vi "Temperature load wafer counts.vi"() -> ()   [LabVIEW 2015, in "VIPM2.lvlib"]
uses:
  VIPM2.lvlib
panel:
  out "Wafer counts":sgl[](array[numeric]) format="%.1f"
  out "ChipIDs":u16[](array[numeric]) format="%04x"
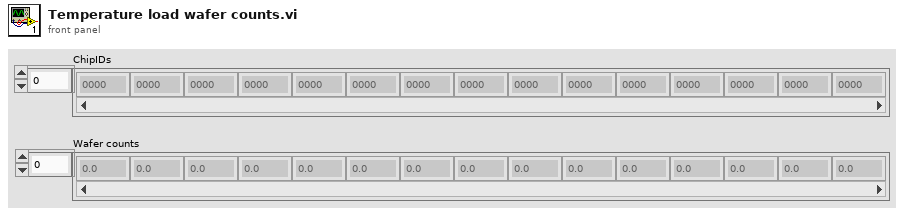
[diagram p1: front panel]
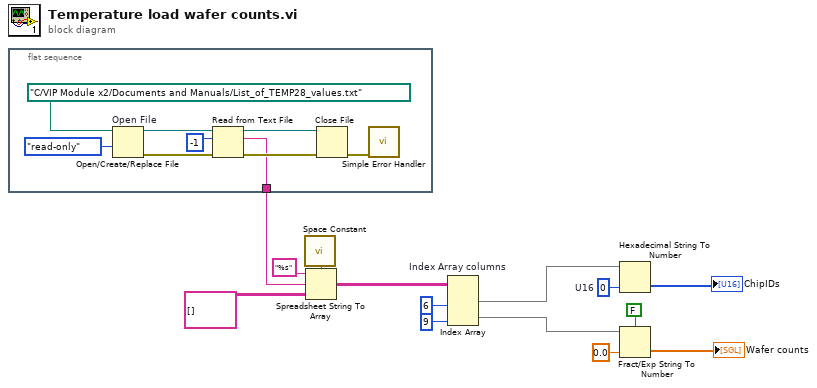
[diagram p0: block diagram]
diagram:
  w6 = u16 0  # U16
  n1 = flat-sequence {
    tunnel: [w15] -> w14
    frame #0 {
      n2 = Open/Create/Replace File "Open File"(file path (use dialog)=path "C:/VIP Module x2/Documents and Manuals/List_of_TEMP28_values.txt", access (0:read/write)=enum16{"read/write", "read-only", "write-only"}."read-only") -> (refnum out=w21:refnum<file>, error out=w19:errorcluster)  [unwired: 4 in, 1 out]
      n3 = Read from Text File(file (use dialog)=w21, count=-1, error in=w19) -> (refnum out=w17:refnum<file>, text=w15:string, error out=w18:errorcluster)  [unwired: 1 in, 1 out]
      n4 = Close File(refnum=w17, error in=w18) -> (error out=w16:errorcluster)  [unwired: 1 out]
      n5 = call <vilib>:"Simple Error Handler.vi"("error in (no error)"=w16) -> ()  [unwired: 4 in, 5 out]
    }
  }
  n6 = call <vilib>:"Space Constant.vi"() -> ("String"=w11:string)
  n7 = Spreadsheet String To Array(delimiter (Tab)=w11, format string="%s", spreadsheet string=w14, array type (2D Dbl)=string[][] []) -> (array=w10:string[][])
  n8 = Index Array "Index Array columns"(array=w10, index (col) #1=6 ("disabled index (col)"), index (col) #2=9 ("index (col)")) -> (element #1=w7:string[], element #2=w4:string[])  [unwired: 2 in]
  n9 = Hexadecimal String To Number(string=w7, default (0uL)=w6) -> (number=→"ChipIDs":u16[])  [unwired: 1 in, 1 out]
  n10 = Fract/Exp String To Number(use system decimal point (T)=FALSE, string=w4, default (0 dbl)=sgl 0.0 ("default (0 DBL)")) -> (number=→"Wafer counts":sgl[])  [unwired: 1 in, 1 out]
